vi "Slide Control  Position.vi"(6 "Direction":enum16{"Right", "Left", "Down", "Up"}(ring), 8 "error in":errorcluster, 11 "Ctl Refnum":refnum<vi>) -> (0 "error out":errorcluster)   [LabVIEW 2018]
doc: "使Control或Indicator做出滑動效果"
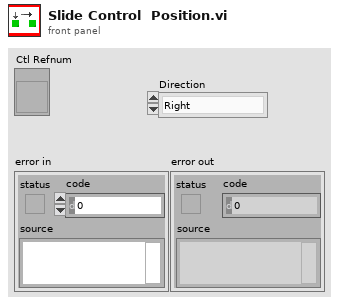
[diagram p1: front panel]
types:
  T1 = typedef "LVPositionTypeDef.ctl" = cluster{"Left":i32, "Top":i32}
  T2 = typedef "LVBoundsTypeDef.ctl" = cluster{"Width":u32, "Height":u32}
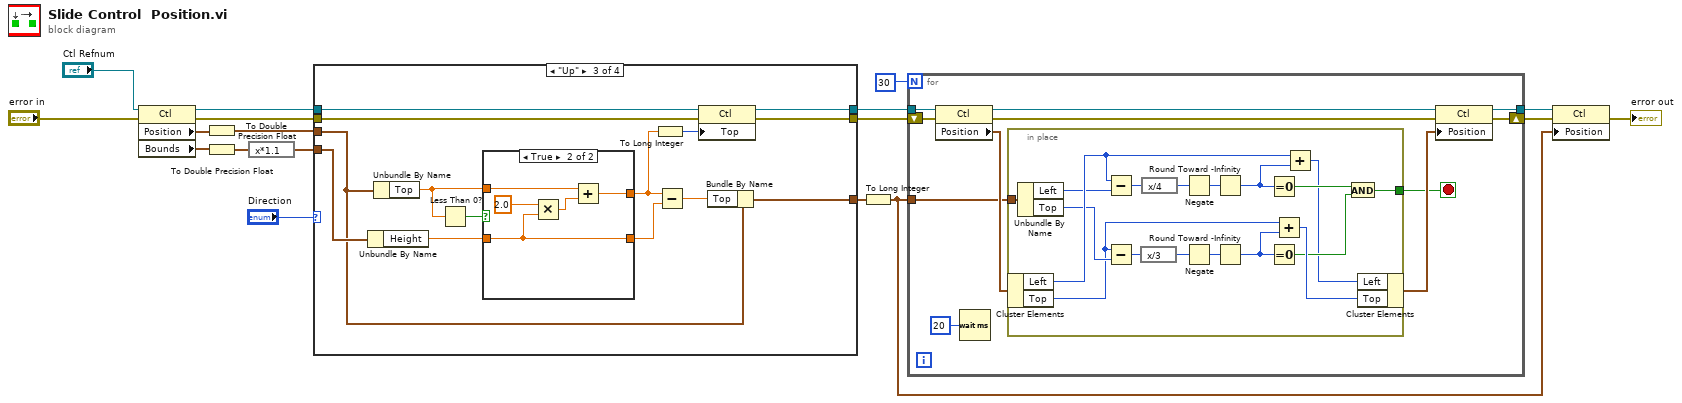
[diagram p0: block diagram]
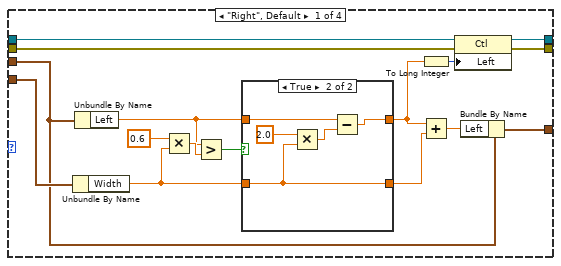
[diagram p2: hidden frame]
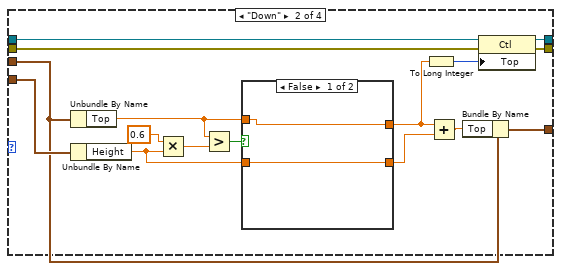
[diagram p4: hidden frame]
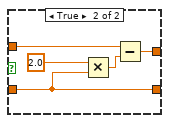
[diagram p5: hidden frame]
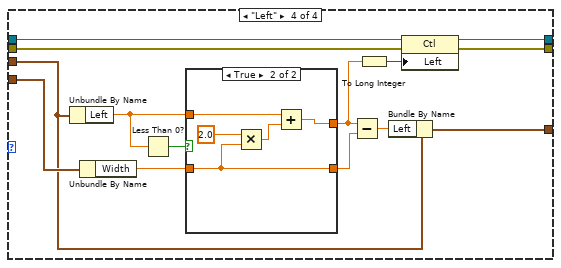
[diagram p7: hidden frame]
diagram:
  n1 = property on="Property Node" class="Ctl"(reference="Ctl Refnum", error in="error in") -> (reference out=w16:refnum<vi>, error out=w14:errorcluster, "Position"=w6:T1, "Bounds"=w8:T2)
  n2 = To Double Precision Float(number=w6) -> (double precision float=w5:cluster{"Left":dbl, "Top":dbl})
  n3 = To Double Precision Float(number=w8) -> (double precision float=w7:cluster{"Width":dbl, "Height":dbl})
  n4 = expression code="x*1.1"(w7) -> (w9:cluster{"Width":dbl, "Height":dbl})
  n5 = case shown="\"Up\"" "Direction" {
    tunnel: w5 -> [w20 w51 w67 w89]
    tunnel: w9 -> [w34 w57 w78 w99]
    tunnel: [w19 w56 w77 w98] -> w4
    tunnel: w16 -> [w33 w55 w76 w97]
    tunnel: [w32 w54 w75 w96] -> w15
    tunnel: w14 -> [w31 w53 w74 w95]
    tunnel: [w30 w52 w73 w94] -> w13
    frame "Right", Default {
      n6 = Unbundle By Name(w34) -> ("Width"=w24:dbl)
      n7 = Unbundle By Name(w20) -> ("Left"=w26:dbl)
      n8 = Multiply(x=0.6, y=w24) -> (x*y=w29:dbl)
      n9 = Greater?(x=w26, y=w29) -> (0:w27:bool)
      n10 = case shown="True" w27 {
        tunnel: w26 -> [w36 w39]
        tunnel: [w36 w38] -> w22
        tunnel: w24 -> [w35 w37]
        tunnel: [w35 w37] -> w23
        frame False {
        }
        frame True {
          n11 = Multiply(x=2.0 ("y"), y=w37) -> (x*y=w41:dbl)
          n12 = Subtract(x=w39, y=w41) -> (x-y=w38:dbl)
        }
      }
      n13 = To Long Integer(number=w22) -> (32bit integer=w21:i32)
      n14 = Add(x=w22, y=w23) -> (x+y=w25:dbl)
      n15 = property on="Property Node" class="Ctl"(reference=w33, error in=w31, "Left"=w21) -> (reference out=w32:refnum<vi>, error out=w30:errorcluster)
      n16 = Bundle By Name(cluster=w20, "Left"=w25) -> (w19:cluster{"Left":dbl, "Top":dbl})
    }
    frame "Down" {
      n17 = Unbundle By Name(w51) -> ("Top"=w44:dbl)
      n18 = Unbundle By Name(w57) -> ("Height"=w43:dbl)
      n19 = Multiply(x=0.6, y=w43) -> (x*y=w50:dbl)
      n20 = Greater?(x=w44, y=w50) -> (0:w48:bool)
      n21 = case shown="False" w48 {
        tunnel: w43 -> [w58 w60]
        tunnel: w44 -> [w59 w62]
        tunnel: [w59 w61] -> w46
        tunnel: [w58 w60] -> w47
        frame False {
        }
        frame True {
          n22 = Multiply(x=2.0 ("y"), y=w60) -> (x*y=w64:dbl)
          n23 = Subtract(x=w62, y=w64) -> (x-y=w61:dbl)
        }
      }
      n24 = To Long Integer(number=w46) -> (32bit integer=w45:i32)
      n25 = Add(x=w46, y=w47) -> (x+y=w42:dbl)
      n26 = Bundle By Name(cluster=w51, "Top"=w42) -> (w56:cluster{"Left":dbl, "Top":dbl})
      n27 = property on="Property Node" class="Ctl"(reference=w55, error in=w53, "Top"=w45) -> (reference out=w54:refnum<vi>, error out=w52:errorcluster)
    }
    frame "Up" {
      n28 = Unbundle By Name(w78) -> ("Height"=w71:dbl)
      n29 = Unbundle By Name(w67) -> ("Top"=w69:dbl)
      n30 = Less Than 0?(x=w69) -> (x < 0?=w72:bool)
      n31 = case shown="True" w72 {
        tunnel: w71 -> [w79 w81]
        tunnel: w69 -> [w80 w83]
        tunnel: [w80 w82] -> w66
        tunnel: [w79 w81] -> w68
        frame False {
        }
        frame True {
          n32 = Multiply(x=2.0 ("y"), y=w81) -> (x*y=w85:dbl)
          n33 = Add(x=w83, y=w85) -> (x+y=w82:dbl)
        }
      }
      n34 = To Long Integer(number=w66) -> (32bit integer=w65:i32)
      n35 = Subtract(x=w66, y=w68) -> (x-y=w70:dbl)
      n36 = property on="Property Node" class="Ctl"(reference=w76, error in=w74, "Top"=w65) -> (reference out=w75:refnum<vi>, error out=w73:errorcluster)
      n37 = Bundle By Name(cluster=w67, "Top"=w70) -> (w77:cluster{"Left":dbl, "Top":dbl})
    }
    frame "Left" {
      n38 = Unbundle By Name(w89) -> ("Left"=w91:dbl)
      n39 = Unbundle By Name(w99) -> ("Width"=w92:dbl)
      n40 = Less Than 0?(x=w91) -> (x < 0?=w93:bool)
      n41 = case shown="True" w93 {
        tunnel: w92 -> [w100 w102]
        tunnel: w91 -> [w101 w104]
        tunnel: [w101 w103] -> w87
        tunnel: [w100 w102] -> w88
        frame False {
        }
        frame True {
          n42 = Multiply(x=2.0 ("y"), y=w102) -> (x*y=w106:dbl)
          n43 = Add(x=w104, y=w106) -> (x+y=w103:dbl)
        }
      }
      n44 = Subtract(x=w87, y=w88) -> (x-y=w90:dbl)
      n45 = To Long Integer(number=w87) -> (32bit integer=w86:i32)
      n46 = Bundle By Name(cluster=w89, "Left"=w90) -> (w98:cluster{"Left":dbl, "Top":dbl})
      n47 = property on="Property Node" class="Ctl"(reference=w97, error in=w95, "Left"=w86) -> (reference out=w96:refnum<vi>, error out=w94:errorcluster)
    }
  }
  n48 = To Long Integer(number=w4) -> (32bit integer=w3:cluster{"Left":i32, "Top":i32})
  n49 = for {
    N: 30 -> [_]
    tunnel: w15 -> [w115]
    shift-right: [w112] -> w10
    shift-left: w13 -> [w114]
    tunnel: [w110] -> w11
    tunnel: w3 -> [w109]
    stop <- w111 stop-if-true
    n50 = property on="Property Node" class="Ctl"(reference=w115, error in=w114) -> (reference out=w108:refnum<vi>, error out=w113:errorcluster, "Position"=w117:T1)
    n51 = Wait (ms)(milliseconds to wait=u32 20) -> ()  [unwired: 1 out]
    n52 = in-place {
      in-place-border: [w130] -> w111
      in-place-border: w109 -> [w129]
      n53 = in-place-cluster #1(w117) -> ("Left"=w134:i32, "Top"=w119:i32)
      n54 = Unbundle By Name(w129) -> ("Left"=w128:i32, "Top"=w127:i32)
      n55 = Subtract(x=w134, y=w128) -> (x-y=w123:i32)
      n56 = Subtract(x=w119, y=w127) -> (x-y=w121:i32)
      n57 = expression code="x/3"(w121) -> (w120:i32)
      n58 = expression code="x/4"(w123) -> (w122:i32)
      n59 = Negate(x=w122) -> (-x=w125:i32)
      n60 = Negate(x=w120) -> (-x=w124:i32)
      n61 = Round Toward -Infinity(1:w125) -> (0:w135:i32)
      n62 = Round Toward -Infinity(1:w124) -> (0:w118:i32)
      n63 = Equal To 0?(x=w135) -> (x = 0?=w131:bool)
      n64 = Equal To 0?(x=w118) -> (x = 0?=w132:bool)
      n65 = Add(x=w119, y=w118) -> (x+y=w133:i32)
      n66 = Add(x=w134, y=w135) -> (x+y=w126:i32)
      n67 = And(x=w131, y=w132) -> (x .and. y?=w130:bool)
      n68 = in-place-cluster #1("Left"=w126, "Top"=w133) -> (w116:T1)
    }
    n69 = property on="Property Node" class="Ctl"(reference=w108, error in=w113, "Position"=w116) -> (reference out=w110:refnum<vi>, error out=w112:errorcluster)
  }
  n70 = property on="Property Node" class="Ctl"(reference=w11, error in=w10, "Position"=w3) -> (error out=→"error out":errorcluster)  [unwired: 1 out]
